vi "Show Panel Object Actions UI.vi"(8 "Error In":errorcluster, 10 "Panel Objects":refnum<class "Panel Object.lvclass">[](array[class]), 11 "Panel Object Actions UI in":refnum<class "Panel Object Actions UI.lvclass">) -> (0 "Error Out":errorcluster, 3 "Panel Object Actions UI out":refnum<class "Panel Object Actions UI.lvclass">)   [LabVIEW 2017, in "Panel Object Actions UI.lvlib" / "Panel Object Actions UI.lvclass"]
uses:
  Panel Object Actions UI.lvclass
  C:/Program Files (x86)/National Instruments/LabVIEW 2017/vi.lib/ActorFramework/Actor/Actor.lvclass
  Panel Object/Panel Object.lvclass
  <vilib>/ActorFramework/Actor/Actor.lvclass/Actor.ctl
  <vilib>/ActorFramework/Message Enqueuer/Message Enqueuer.lvclass/Message Enqueuer.ctl
  Panel Object Actions UI.lvclass/Panel Object Actions UI.ctl
  <vilib>/ActorFramework/Message Enqueuer/Init from Existing Queue.vi
  <vilib>/ActorFramework/Message Enqueuer/Message Enqueuer.lvclass
  <vilib>/ActorFramework/Actor/Actor.lvclass
  <vilib>/MNProjects/Panel Manager/panel-actors/Source/Panel Actor Messages/Show Panel Msg/Show Panel Msg.lvclass
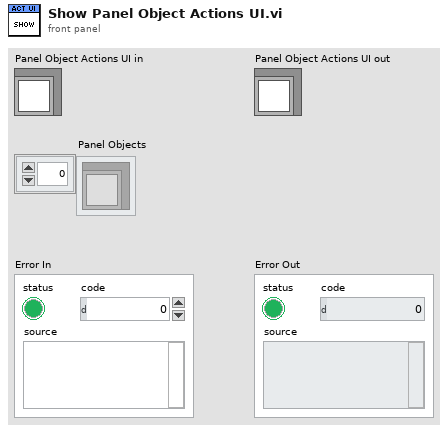
[diagram p1: front panel]
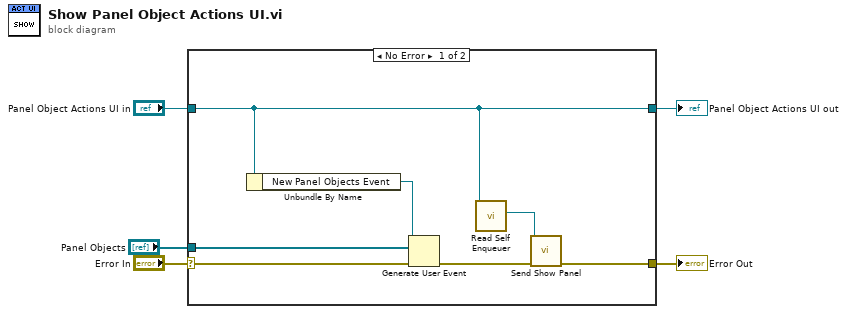
[diagram p0: block diagram]
diagram:
  n1 = case shown="No Error" "Error In" {
    selector: "Error In" -> [w9 w14]
    tunnel: [w8 w14] -> w2
    tunnel: [w6 w13] -> w4
    tunnel: "Panel Object Actions UI in" -> [w6 w13]
    tunnel: "Panel Objects" -> [w7 _]
    frame No Error {
      n2 = Unbundle By Name(w6) -> ("New Panel Objects Event"=w12:refnum<user-event>)
      n3 = Generate User Event(user event=w12, event data cluster=w7, error in=w9) -> (error out=w11:errorcluster)  [unwired: 1 in, 1 out]
      n4 = call <vilib>:"Read Self Enqueuer.vi"("Actor"=w6) -> ("Self Enqueuer"=w10:refnum<class "Message Enqueuer.lvclass">)  [unwired: 10 in]
      n5 = call <vilib>:"Send Show Panel.vi"("error in (no error)"=w11, "Message Enqueuer in"=w10) -> ("error out"=w8:errorcluster)  [unwired: 8 in, 1 out]
    }
    frame Error {
    }
  }
  "Panel Object Actions UI out" <- w4
  "Error Out" <- w2
